vi "MoM.vi"(2 "outputterm default (0)":u8, 3 "output when no consequence (0)":u16(ring) items=["last result", "Default"], 4 "fullfilment consequence":dbl[](array[numeric])=[0.0, 0.25, 0.75] step=0.01 format="%.2f", 5 "consequence":T1(array[cluster])=[{"ling.var."="out", "x-min"=-1.0, "x-max"=1.0, "setarray"=[{"linguistic term"="NEo", "color"=16711680, "points"=[-1.0, -1.0, -1.0, 0.0]}, {"linguistic term"="ZEo", "color"=255, "points"=[-1.0, 0.0, 0.0, 1.0]}, {"linguistic term"="POo", "color"=26214, "points"=[0.0, 1.0, 1.0, 1.0]}]}] {"x-min" format="%.2f"; "x-max" format="%.2f"; "setarray"."points" min=-1.0 max=1.0 step=0.10000000149011612 format="%.2f"}) -> (0 "output assessment":string, 1 "controller output":dbl format="%.2f")   [LabVIEW 2017, in "NI_fuzzy logic.lvlib"]
doc: "Defuzzify (Mean-of-Maximum)\nThis VI is used to find the plausiblest result for processing.\noutput : typ. value of consequenceterm with the highest fullfilment \nOutput : Analog value for controlling\nInputs : -consequencearray\n - fullfillment of each term ...\n - output when no consequence term is firering\n (0: last value , 1: Defaultvalue)"
uses:
  <vilib>/addons/control/fuzzy/NI_fuzzy logic.lvlib
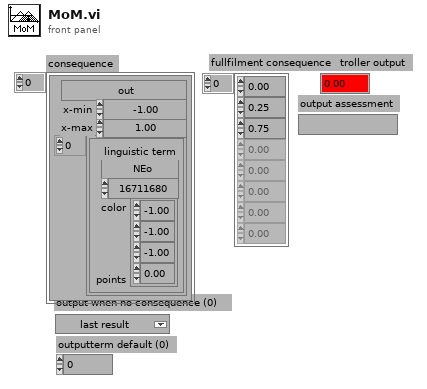
[diagram p1: front panel]
types:
  T1 = cluster{"ling.var.":string, "x-min":dbl, "x-max":dbl, "setarray":cluster{"linguistic term":string, "color":u32, "points":dbl[]}[]}[]
  T2 = cluster{"ling.var.":string, "x-min":dbl, "x-max":dbl, "setarray":cluster{"linguistic term":string, "color":u32, "points":dbl[]}[]}
  T3 = cluster{"linguistic term":string, "color":u32, "points":dbl[]}[]
  T4 = cluster{"linguistic term":string, "color":u32, "points":dbl[]}
  T5 = cluster{"points[0]":dbl, "points[1]":dbl, "points[2]":dbl, "points[3]":dbl}
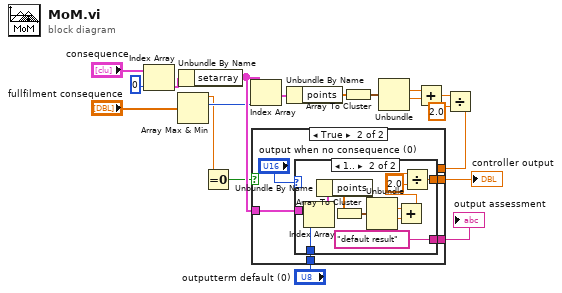
[diagram p0: block diagram]
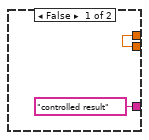
[diagram p2: hidden frame]
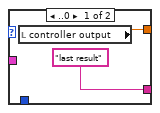
[diagram p3: hidden frame]
diagram:
  n1 = Index Array(array="consequence", index=0) -> (element=w3:T2)
  n2 = Array Max & Min(array="fullfilment consequence") -> (max value=w11:dbl, max index (indices)=w15:i32)  [unwired: 2 out]
  n3 = Unbundle By Name(w3) -> ("setarray"=w16:T3)
  n4 = Equal To 0?(x=w11) -> (x = 0?=w12:bool)
  n5 = Index Array(array=w16, index=w15) -> (element=w9:T4)
  n6 = Unbundle By Name(w9) -> ("points"=w10:dbl[])
  n7 = Array To Cluster(array=w10) -> (cluster=w4:T5)
  n8 = Unbundle(w4) -> ("points[1]"=w5:dbl, "points[2]"=w6:dbl)  [unwired: 2 out]
  n9 = Add(x=w5, y=w6) -> (x+y=w7:dbl)
  n10 = Divide(x=w7, y=2.0) -> (x/y=w13:dbl)
  n11 = case shown="True" w12 {
    tunnel: w13 -> [w21 _]
    tunnel: [w21 w25] -> w14
    tunnel: w16 -> [_ w24]
    tunnel: "outputterm default (0)" -> [_ w23]
    tunnel: ["controlled result" w22] -> w1
    frame False {
    }
    frame True {
      n12 = case shown="1.." "output when no consequence (0)" {
        tunnel: [w28 w31] -> w25
        tunnel: w24 -> [_ w39]
        tunnel: w23 -> [_ w30]
        tunnel: ["last result" "default result"] -> w22
        frame ..0 {
          n13 = local read "controller output"() -> (w28:dbl)
        }
        frame 1.. {
          n14 = Index Array(array=w39, index=w30) -> (element=w38:T4)
          n15 = Unbundle By Name(w38) -> ("points"=w37:dbl[])
          n16 = Array To Cluster(array=w37) -> (cluster=w36:T5)
          n17 = Unbundle(w36) -> ("points[1]"=w35:dbl, "points[2]"=w34:dbl)  [unwired: 2 out]
          n18 = Add(x=w35, y=w34) -> (x+y=w33:dbl)
          n19 = Divide(x=w33, y=2.0) -> (x/y=w31:dbl)
        }
      }
    }
  }
  "controller output" <- w14
  "output assessment" <- w1
